vi "RT Main R3.vi"() -> ()   [LabVIEW 2018]
uses:
  <vilib>/rvi/interface/nirviOpenFPGA/nirviOpenFPGA.xnode
  Type Defs/Measurement States.ctl
  Support Libraries/Message Queue/Message Queue.lvlib
  Global Variables/RT Loop Stop.vi
  <vilib>/rvi/interface/nirviReadWriteControl/nirviReadWriteControl.xnode
  Type Defs/Control Mode.ctl
  <vilib>/rvi/interface/nirviMethod/nirviMethod.xnode
  <vilib>/rvi/interface/nirviMethod/StockFPGA_InlinedMethodWaitForSingleIRQ.vi
  <vilib>/FPGAPlugInAG/Dynamic/niLvFpga_WaitOnIrq_Dynamic.vi
  <vilib>/FPGAPlugInAG/Dynamic/niLvFpga_AcknowledgeIrq_Dynamic.vi
  NiFpgaLv.dll
  <vilib>/Utility/error.llb/Error Cluster From Error Code.vi
  <vilib>/rvi/interface/Simulation/niFpgaSimulationCallBeginRW.vi
  <vilib>/rvi/errors/niLvFpgaAdjustHostInterfaceError.vi
  FPGA Bitfiles/WattBalanceRev1_FPGATarget_FPGAMain_doRdIs9Lwbc.lvbitx
  FPGA/FPGA Main R3 AB JC KV.vi
  <vilib>/FPGAPlugInAG/myRIO-1900/niLvFpga_Open_myRIO-1900.vi
  <vilib>/rvi/interface/common/dynamic/niFpgaDynamicAddResources.vi
panel:
  out "IRQ Timeout":bool
  in  "Measure BL":bool
  out "data out":u16[][](array[numeric])
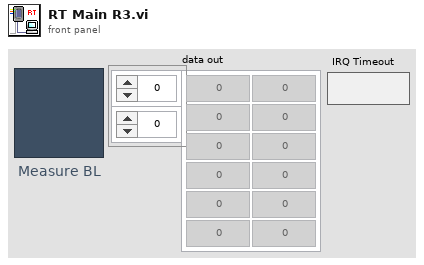
[diagram p1: front panel]
types:
  T1 = typedef "Measurement States.ctl" = enum16{"Idle", "Initialize", "Measure", "Collect Data", "Calculate", "Close"}
  T2 = typedef "Control Mode.ctl" = enum16{"Start Velocity", "Velocity", "End Velocity", "Displacement", "Manual"}
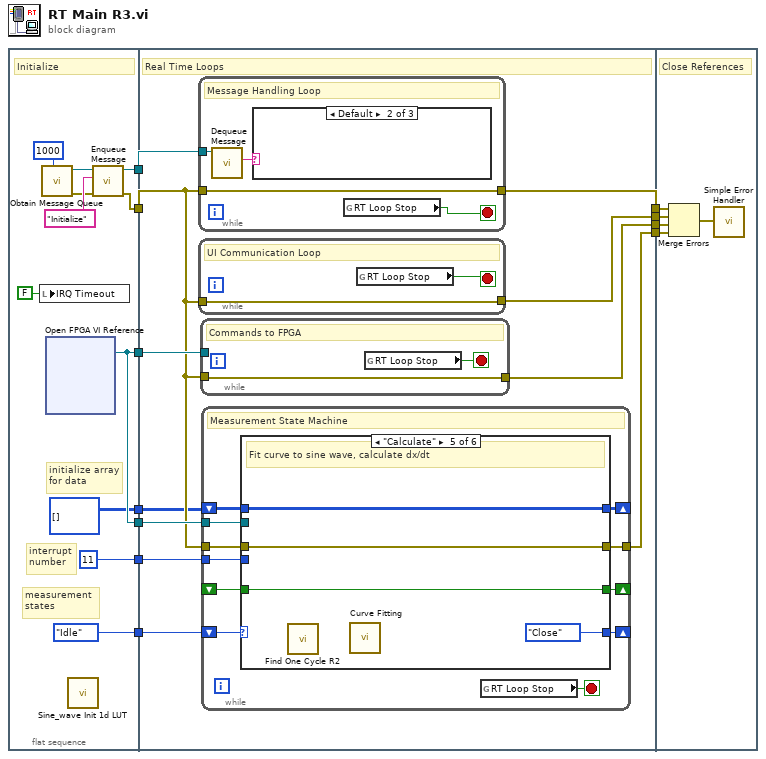
[diagram p0: block diagram]
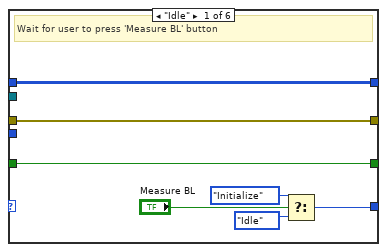
[diagram p4: hidden frame]
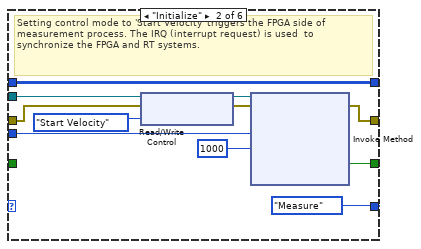
[diagram p5: hidden frame]
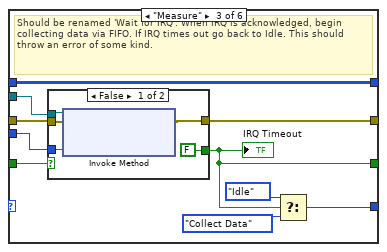
[diagram p6: hidden frame]
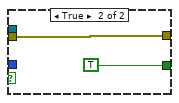
[diagram p7: hidden frame]
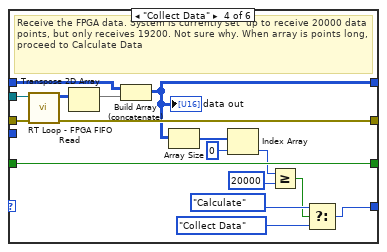
[diagram p8: hidden frame]
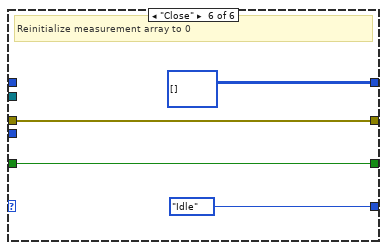
[diagram p9: hidden frame]
diagram:
  n1 = flat-sequence {
    tunnel: [w16] -> w11
    tunnel: [w15] -> w10
    tunnel: [Measurement_States."Idle" ("Enum")] -> w8
    tunnel: [w18] -> w7
    tunnel: [w15] -> w3
    tunnel: [11 ("IRQ Number(s)")] -> w2
    tunnel: [u16[][] []] -> w1
    tunnel: w11 -> [w25]
    tunnel: w10 -> [w30]
    tunnel: [w33] -> w9
    tunnel: w8 -> [w32]
    tunnel: w7 -> [w31]
    tunnel: [w29] -> w6
    tunnel: [w28] -> w5
    tunnel: [w27] -> w4
    tunnel: w3 -> [w26]
    tunnel: w2 -> [w24]
    tunnel: w1 -> [w23]
    tunnel: w9 -> [w112]
    tunnel: w6 -> [w115]
    tunnel: w5 -> [w114]
    tunnel: w4 -> [w113]
    frame #0 {
      # "measurement\nstates"
      # "interrupt\nnumber"
      # "initialize array\nfor data"
      # "Initialize"
      n2 = local write "IRQ Timeout"(FALSE ("IRQ Timeout")) -> ()
      n3 = call "Obtain Message Queue.vi"("max queue size (-1, unlimited)"=1000) -> ("error out"=w17:errorcluster, "Message Queue"=w20:refnum<queue>)  [unwired: 9 in]
      n4 = xnode "Open FPGA VI Reference"() -> ("FPGA VI Reference Out"=w15:refnum<k20>)  [unwired: 2 in, 1 out]
      n5 = call "Sine_wave Init 1d LUT.vi"() -> ()  [unwired: 11 in, 1 out]
      n6 = call "Enqueue Message.vi"("error in (no error)"=w17, "Message"="Initialize", "Message Queue"=w20) -> ("error out"=w16:errorcluster, "dup Message Queue"=w18:refnum<queue>)  [unwired: 7 in]
    }
    frame #1 {
      # "Real Time Loops"
      n7 = while {
        tunnel: w25 -> [w39]
        tunnel: w31 -> [w41]
        tunnel: [w39] -> w29
        stop <- w38 stop-if-true
        # "Message Handling Loop"
        n8 = call "Dequeue Message.vi"("Message Queue"=w41) -> ("Message"=w40:string)  [unwired: 7 in, 3 out]
        n9 = case shown="Default" w40 {
          frame "Initialize" {
          }
          frame Default {
          }
          frame "Exit" {
          }
        }
        n10 = global read "RT Loop Stop.vi" "RT Loop Stop"() -> (w38:bool)
      }
      n11 = while {
        tunnel: [w35] -> w27
        tunnel: w25 -> [w35]
        stop <- w34 stop-if-true
        # "UI Communication Loop"
        n12 = global read "RT Loop Stop.vi" "RT Loop Stop"() -> (w34:bool)
      }
      n13 = while {
        tunnel: w30 -> [_]
        tunnel: w25 -> [w36]
        tunnel: [w36] -> w28
        stop <- w37 stop-if-true
        # "Commands to FPGA"
        n14 = global read "RT Loop Stop.vi" "RT Loop Stop"() -> (w37:bool)
      }
      n15 = while {
        tunnel: w25 -> [w48]
        tunnel: [w45] -> w33
        shift-right: [w50] -> _
        shift-left: w32 -> [w52]
        tunnel: w26 -> [w49]
        shift-right: [w47] -> _
        shift-left: w23 -> [w46]
        tunnel: w24 -> [w44]
        shift-right: [w43] -> _
        shift-left: _ -> [w42]
        stop <- w51 stop-if-true
        # "Measurement State Machine"
        n16 = case shown="\"Calculate\"" w52 {
          tunnel: [w57 Measurement_States."Measure" ("Enum") w72 w89 Measurement_States."Close" ("Enum") Measurement_States."Idle" ("Enum")] -> w50
          tunnel: w49 -> [_ w69 w71 w96 _ _]
          tunnel: w48 -> [w54 w67 w79 w103 w105 w110]
          tunnel: [w55 w68 w80 w97 w106 u16[][] []] -> w47
          tunnel: w46 -> [w55 w68 w80 w102 w106 _]
          tunnel: [w54 w64 w73 w101 w105 w110] -> w45
          tunnel: w44 -> [_ w62 w78 _ _ _]
          tunnel: [w53 w61 w74 w98 w104 w109] -> w43
          tunnel: w42 -> [w53 _ w77 w98 w104 w109]
          frame "Idle" {
            # "Wait for user to press 'Measure BL' button"
            n17 = Select(t=Measurement_States."Initialize" ("Enum"), s="Measure BL", f=Measurement_States."Idle" ("Enum")) -> (s? t:f=w57:T1)
          }
          frame "Initialize" {
            # "Setting control mode to 'Start Velocity' triggers the FPGA side of measurement process. The IRQ (interrupt request) is used  to synchronize the FPGA and RT systems."
            n18 = xnode "Read/Write Control"("FPGA VI Reference In"=w69, "error in"=w67, "Control Mode"=Control_Mode."Start Velocity") -> ("FPGA VI Reference Out"=w66:refnum<k20>, "error out"=w65:errorcluster)
            n19 = xnode "Invoke Method"("FPGA VI Reference In"=w66, "error in"=w65, "IRQ Number(s)"=w62, "Timeout (ms)"=1000) -> ("error out"=w64:errorcluster, "Timed Out"=w61:bool)  [unwired: 2 out]
          }
          frame "Measure" {
            # "Should be renamed 'Wait for IRQ'. When IRQ is acknowledged, begin collecting data via FIFO. If IRQ times out go back to Idle. This should throw an error of some kind."
            n20 = case shown="False" w77 {
              tunnel: w71 -> [w85 _]
              tunnel: w79 -> [w84 w86]
              tunnel: w78 -> [w83 _]
              tunnel: [FALSE TRUE] -> w74
              tunnel: [w81 w86] -> w73
              frame False {
                n21 = xnode "Invoke Method"("FPGA VI Reference In"=w85, "error in"=w84, "IRQ Number(s)"=w83) -> ("error out"=w81:errorcluster)  [unwired: 1 out]
              }
              frame True {
              }
            }
            "IRQ Timeout" <- w74
            n22 = Select(t=Measurement_States."Idle" ("Enum"), s=w74, f=Measurement_States."Collect Data" ("Enum")) -> (s? t:f=w72:T1)
          }
          frame "Collect Data" {
            # "Receive the FPGA data. System is currently set  up to receive 20000 data points, but only receives 19200. Not sure why. When array is points long, proceed to Calculate Data"
            n23 = call "RT Loop - FPGA FIFO Read.vi"("error in (no error)"=w103, "FPGA VI Reference In"=w96) -> ("error out"=w101:errorcluster, "Data Out"=w100:u16[][])  [unwired: 8 in]
            n24 = Transpose 2D Array(2D array=w100) -> (transposed array=w99:u16[][])
            n25 = Build Array (concatenate)(w102, w99) -> (w97:u16[][])
            "data out" <- w97
            n26 = Array Size(array=w97) -> (size(s)=w94:i32[])
            n27 = Index Array(array=w94, index=0) -> (element=w92:i32)
            n28 = Greater Or Equal?(x=w92, y=20000) -> (x >= y?=w88:bool)
            n29 = Select(t=Measurement_States."Calculate" ("Enum"), s=w88, f=Measurement_States."Collect Data" ("Enum")) -> (s? t:f=w89:T1)
          }
          frame "Calculate" {
            # "Fit curve to sine wave, calculate dx/dt"
            n30 = call "Find One Cycle R2.vi"() -> ()  [unwired: 10 in, 2 out]
            n31 = call "Curve Fitting"() -> ()  [unwired: 7 in, 5 out]
          }
          frame "Close" {
            # "Reinitialize measurement array to 0"
          }
        }
        n32 = global read "RT Loop Stop.vi" "RT Loop Stop"() -> (w51:bool)
      }
    }
    frame #2 {
      # "Close References"
      n33 = Merge Errors(w115, w113, w114, w112) -> (w116:errorcluster)
      n34 = call <vilib>:"Simple Error Handler.vi"("error in (no error)"=w116) -> ()  [unwired: 4 in, 5 out]
    }
  }
